vi "FPGA_HoppingScan_MultiRegion.vi"() -> ()   [LabVIEW 2024]
uses:
  <vilib>/Platform/TimedLoop/XDataNode/timing_clust.ctl
  <vilib>/Platform/TimedLoop/XDataNode/nitl_modes.ctl
  <vilib>/Platform/TimedLoop/XDataNode/wakeup.ctl
  <vilib>/rvi/FXPMathLib/FxpDiv/subVIs/nifxpmath_Div_SimConfig.ctl
  <vilib>/rvi/Emulation/niFpgaSctlEmulationGetInTimedLoop.vi
  <vilib>/rvi/Emulation/niFpgaProcessEmulError.vi
  <vilib>/rvi/eio/common/nirviEmuTemplateMethod_errors.vi
  <vilib>/rvi/Memory/Memory_Emulation/nirvimemoryFastEmulation.vi
  <vilib>/rvi/Memory/Memory_Emulation/nirvimemoryEmulation.vi
  <vilib>/rvi/Emulation/niFpgaEmulationIsFPGAContextNoSignature.vi
  <vilib>/rvi/DataTransferAndStorage/Container/Common/niFpgaContainerGetUniqueNameForEmu.vi
  <vilib>/rvi/errors/nirviReportUnexpectedCaseInternalError (U32).vi
  <vilib>/rvi/Emulation/niFpgaEmulationReportErrorSimple.vi
  <vilib>/rvi/Emulation/niFpgaGetClockAttributes.vi
  <vilib>/rvi/Emulation/niFpgaCriticalErrorInLSC.vi
  <vilib>/rvi/Memory/Memory_Emulation/niFpgaMemoryEmulationCacheClearOnFirstRun.vi
  <vilib>/rvi/Memory/Memory_Emulation/nirvimemoryEmulationManagerCache_MakeExclusive.vi
  <vilib>/rvi/Memory/Memory_Emulation/niFpgaMemoryEmulationValidateCache.vi
  <vilib>/rvi/Memory/Memory_Emulation/nirvimemoryEmulationManagerCache_InsertValue.vi
  <vilib>/Utility/error.llb/Clear Errors.vi
  <vilib>/rvi/Memory/Memory_Emulation/nirvimemoryEmulationManagerCache_ReleaseExclusive.vi
  <vilib>/rvi/Memory/Memory_Emulation/nirvimemoryEmulationManagerCache_GetValue.vi
  <vilib>/rvi/Memory/Memory_Emulation/nirvimemoryEmulationManagerCache_SetValue.vi
  <vilib>/rvi/FIFO/Fifo_Resource/nirvififoEmulationSetSize.vi
  <vilib>/rvi/FIFO/Fifo_Resource/nirviFifoEmulationQueueMgr.vi
  <instcachedir>/0/nirviFifoEmulationQueueMgr_E5CAEC123FF24DC58D834DCA3CDAA9B5.lvgen/nirviFifoEmulationQueueMgr_E5CAEC123FF24DC58D834DCA3CDAA9B5_001.vi
  <vilib>/rvi/errors/niFpgaSetErrorForExecOnDevCompSimple.vi
  <vilib>/rvi/eio/common/nirviEmuReportErrorAndStop.vi
  <vilib>/rvi/FIFO/Fifo_Resource/nirvififoEmulationCreateLock.vi
  <vilib>/rvi/FIFO/Fifo_Resource/nirvififoEmulationObtainLock.vi
  <vilib>/rvi/FIFO/Fifo_Resource/nirvififoEmulationReleaseLock.vi
  <vilib>/rvi/occurrence/nirviWaitOnOccurrenceBase.vi
  <vilib>/rvi/errors/nirviReportUnexpectedCaseInternalError.vi
  <vilib>/eio/utilities/niEioResolveVilibRelativePath.vi
  <vilib>/rvi/interface/RandomDataEmulation/niFpgaRandomDataHandleErrors.vi
  <vilib>/rvi/FXPMathLib/FxpDiv/simVIs/DllFxpDivTemp_sub.vi
  <vilib>/rvi/FIFO/Fifo_Resource/nirvififoEmulationDetermineInputValidOut.vi
  <vilib>/eio/EIONode/EIONode.xnode
  <vilib>/rvi/DataTransferAndStorage/Container/XNode/niFpgaContainer.xnode
  <vilib>/platform/TimedLoop/XDataNode/XDataNode.xnode
  <vilib>/rvi/DataTransferAndStorage/Register/Emulation/niFpgaRegisterEmulation.vi
  <vilib>/rvi/FIFO/Fifo_Resource/nirvififoEmulationGetNumberOfElementsToRead.vi
  <vilib>/rvi/FIFO/Fifo_Resource/nirvififoEmulationRead.vi
  <vilib>/rvi/interface/RandomDataEmulation/nirviRandomDataFpgaReadWriteTemplate.vi
  <vilib>/rvi/FXPMathLib/FxpSub/XNode/nifxpmath_Sub.xnode
  <vilib>/rvi/FXPMathLib/FxpAdd/XNode/nifxpmath_Add.xnode
  <vilib>/rvi/FXPMathLib/FxpMul/XNode/nifxpmath_Multiplier.xnode
  <vilib>/rvi/FXPMathLib/FxpDiv/XNode/nifxpmath_Div.xnode
  <vilib>/rvi/FIFO/Fifo_Resource/nirvififoEmulationWrite.vi
  <vilib>/rvi/FXPMathLib/sim/FxpSim.dll
  <vilib>/Platform/TimedLoop/XDataNode/XDNodeRunTimeDep.lvlib
panel:
  in  "LastScan":bool
  in  "InitScan":bool
  in  "DelayPoints":i32
  in  "Halting Threshold":fxp<+/-,48,16>
  out "point_scanned":u32
  in  "TotalPoints":u32
  in  "RetRate us":i32
  in  "AppRate_NF us":i32
  in  "AppRate_FF us":i32
  in  "Recording Threshold":fxp<+/-,48,16>
  in  "stop":bool
  out "TargetDone?":bool
  out "ScanFinished?":bool
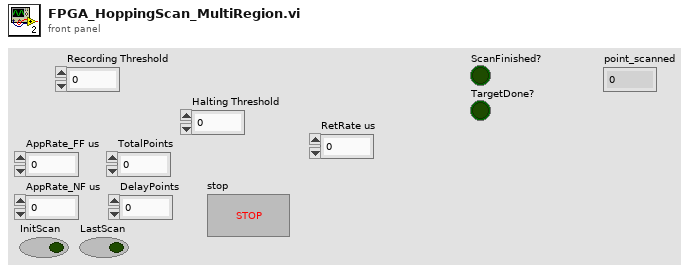
[diagram p1: front panel]
types:
  T1 = typedef "XDNodeRunTimeDep.lvlib/timing_clust.ctl" = cluster{"Expected End [f-1]":u64, "Actual End [f-1]":u64, "Finished Late? [f-1]":bool, "Expected End [i-1]":u64, "Actual End [i-1]":u64, "Finished Late? [i-1]":bool, "Expected Start [i]":u64, "Actual Start [i]":u64, "Expected Start [f]":u64, "Actual Start [f]":u64, "Source Name":string, "Structure Name":string, "Period":i64, "Deadline":i64, "Offset":i64, "Start":i64, "Priority":i32, "Timeout":i32, "Mode":T2, "Wakeup Reason":T3, "Error":errorcluster, "Source Type":string, "Secondary Source Type":string, "Global End Time":u64, "Global Start Time":u64, "Frame Duration":u64, "Iteration Duration":u64, "Assigned CPU":i32, "I/O Scan Engine Mode":u32}
  T2 = typedef "XDNodeRunTimeDep.lvlib/nitl_modes.ctl" = enum32{"No Change", "Process missed periods, maintain original phase", "Discard missed periods, maintain original phase", "Process missed periods, ignore original phase", "Discard missed periods, ignore original phase"}
  T3 = typedef "XDNodeRunTimeDep.lvlib/wakeup.ctl" = enum32{"Normal", "Aborted", "Asynchronous wakeup", "Timing source error", "Timed loop error", "Timeout"}
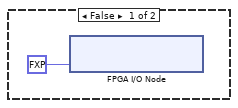
[diagram p2: hidden frame]
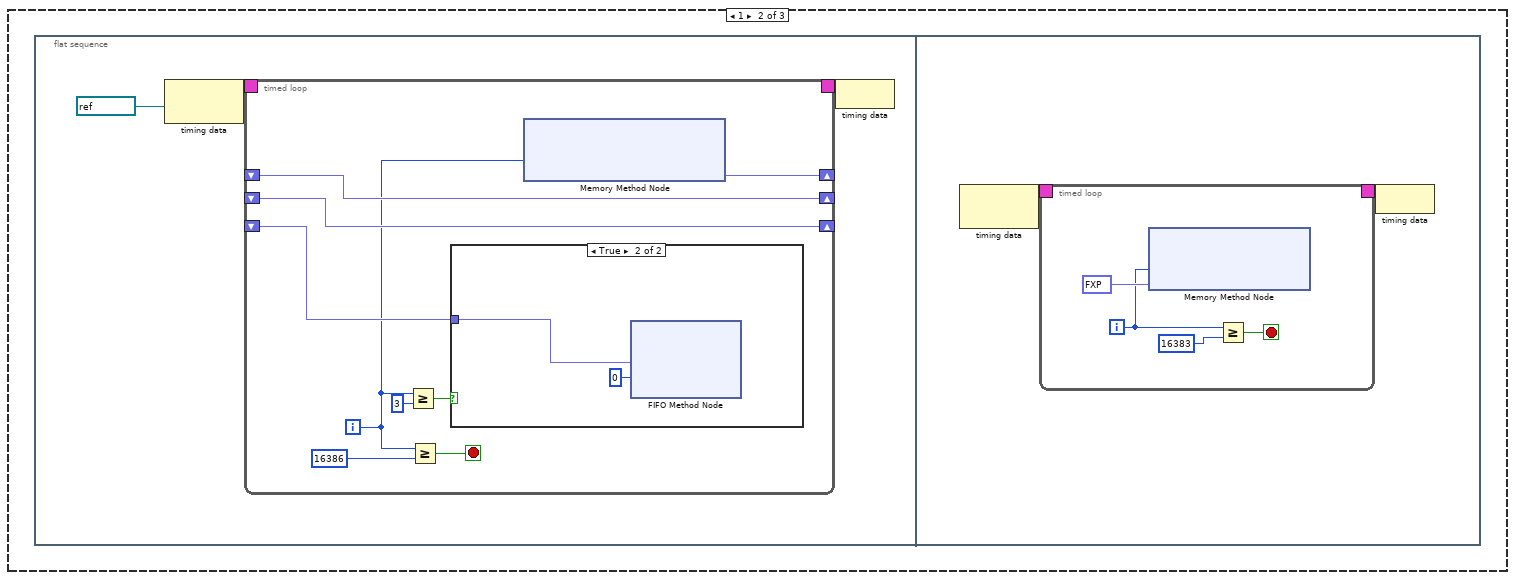
[diagram p5: hidden frame]
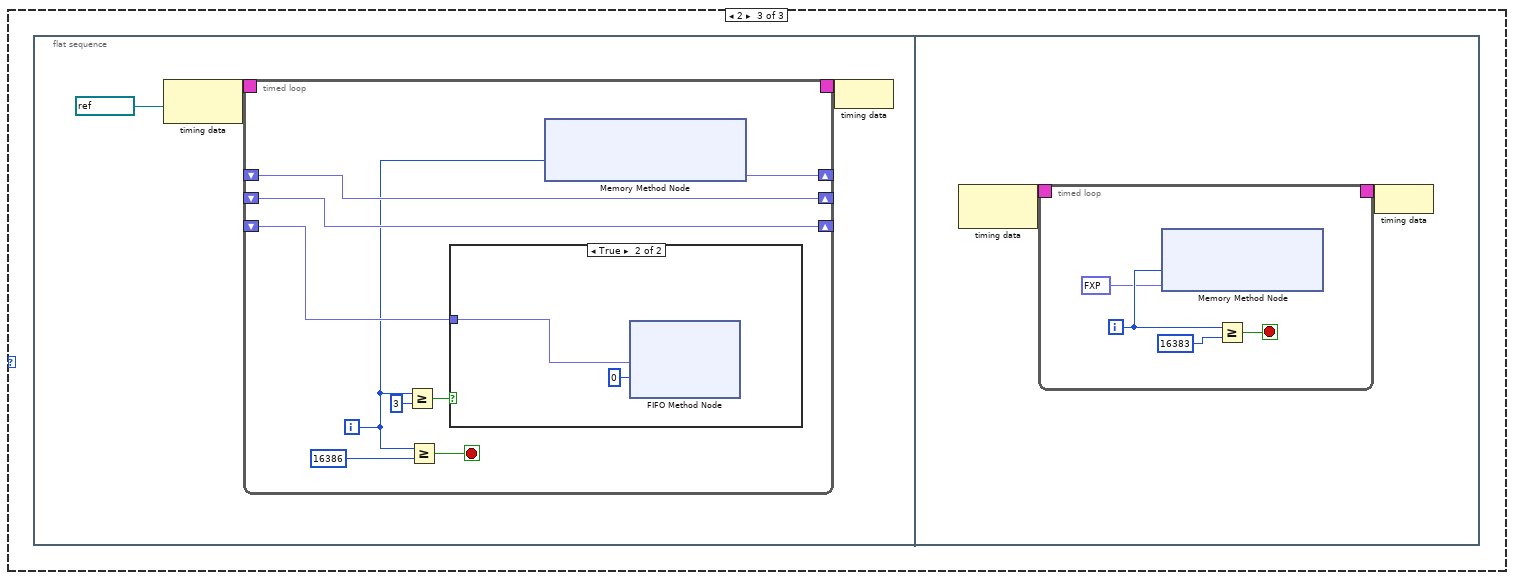
[diagram p7: hidden frame]
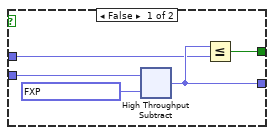
[diagram p14: hidden frame]
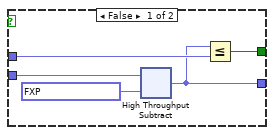
[diagram p15: hidden frame]
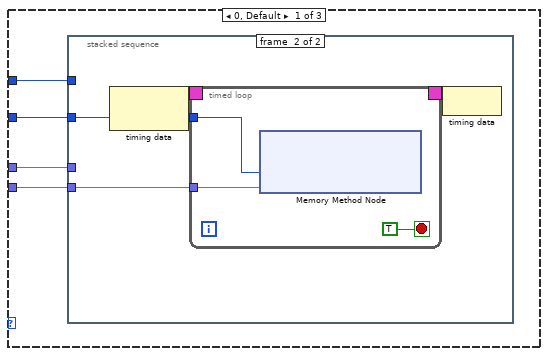
[diagram p17: hidden frame]
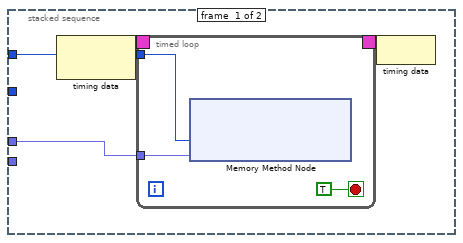
[diagram p18: hidden frame]
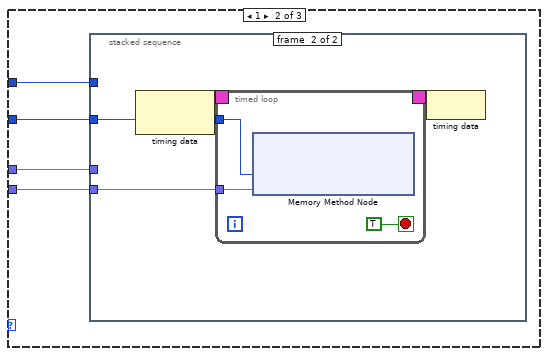
[diagram p19: hidden frame]
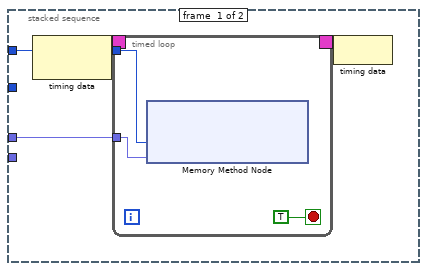
[diagram p20: hidden frame]
diagram:
  n1 = flat-sequence {
    tunnel: [w21] -> w1
    tunnel: w1 -> [w34]
    frame #0 {
      n2 = call "Wait18"("Count(mSec)"=u8 150) -> ()  [unwired: 1 out]
    }
    frame #1 {
      n3 = node-c288() -> (w5:T1)  [unwired: 1 in]
      n4 = timed-loop {
        timing: w5 -> [_]
        timing-out: [_] -> w4
        i -> [w14]
        stop <- w13 stop-if-true
        w16 = fxp<+/-,48,16> -100.0 ("Data")
        n5 = xnode ("Memory Method Node")("Address"=w14, "Data"=w16) -> ()  [unwired: 1 in, 1 out]
        n6 = xnode ("Memory Method Node")("Address"=w14, "Data"=w16) -> ()  [unwired: 1 in, 1 out]
        n7 = xnode ("Memory Method Node")("Address"=w14, "Data"=w16) -> ()  [unwired: 1 in, 1 out]
        n8 = Greater Or Equal?(x=w14, y=16383) -> (x >= y?=w13:bool)
      }
      n9 = case shown="True" "InitScan" {
        frame False {
          n10 = xnode "FPGA I/O Node"("Connector0/AO2"=fxp<+/-,20,5> 0.0 ("Connector0/AO0")) -> ()  [unwired: 1 in, 1 out]
        }
        frame True {
          w10 = fxp<+/-,20,5> 0.0 ("Connector0/AO0")
          n11 = for {
            N: 6 -> [_]
            i -> [w12]
            n12 = xnode ("Memory Method Node")("Address"=w12, "Data"=fxp<+/-,48,16> 0.0) -> ()  [unwired: 1 in, 1 out]
          }
          n13 = xnode "FPGA I/O Node"("Connector0/AO0"=w10, "Connector0/AO1"=w10, "Connector0/AO2"=w10) -> ()  [unwired: 3 in, 3 out]
        }
      }
      n14 = node-c288(w4) -> ()
      "ScanFinished?" <- FALSE
      "TargetDone?" <- FALSE
    }
    frame #2 {
      n15 = Generate Occurrence() -> (w21:refnum<k4>)
      n16 = call "Wait"("Count(mSec)"=u8 50) -> ()  [unwired: 1 out]
    }
    frame #3 {
      n17 = while {
        tunnel: w34 -> [w151]
        stop <- w153 stop-if-true
        n18 = xnode ("Register Read")() -> ("Data"=w154:bool)  [unwired: 1 in, 1 out]
        n19 = xnode ("FIFO Method Node")() -> ("Number of Elements to Read"=w157:u32)  [unwired: 1 in, 1 out]
        n20 = local read "ScanFinished?"() -> (w152:bool)
        n21 = Or(x=w154, y=w152) -> (x .or. y?=w153:bool)
        n22 = Greater Or Equal?(x=w157, y=u32 6) -> (x >= y?=w155:bool)
        n23 = case shown="True" w155 {
          tunnel: w151 -> [_ w158]
          frame False {
          }
          frame True {
            n24 = First Call?() -> (First Call?: T/F=w159:bool)
            n25 = case shown="True" w159 {
              tunnel: w158 -> [_ w160]
              frame False {
              }
              frame True {
                n26 = flat-sequence {
                  tunnel: [w163] -> w161
                  tunnel: w160 -> [w163]
                  tunnel: w161 -> [w164]
                  frame #0 {
                    n27 = call "Wait3"("Count(mSec)"=u8 4) -> ()  [unwired: 1 out]
                  }
                  frame #1 {
                    n28 = Set Occurrence(w164) -> ()
                  }
                }
              }
            }
          }
        }
      }
      n29 = while {
        tunnel: w34 -> [w136]
        stop <- w133 stop-if-true
        n30 = flat-sequence {
          tunnel: ["stop"] -> w138
          tunnel: w136 -> [w140]
          tunnel: [w140] -> w134
          tunnel: w138 -> [w143]
          tunnel: [w143] -> w137
          tunnel: [w142] -> w135
          tunnel: w134 -> [w142]
          tunnel: w137 -> [w147]
          tunnel: w135 -> [w146]
          tunnel: [w145] -> w133
          frame #0 {
            n31 = case shown="True" "stop" {
              tunnel: "stop" -> [_ w141]
              frame False {
              }
              frame True {
                n32 = xnode ("Register Write")("Data"=w141) -> ()  [unwired: 1 in, 1 out]
              }
            }
          }
          frame #1 {
            n33 = call "Wait2"("Count(uSec)"=u8 200) -> ()  [unwired: 1 out]
          }
          frame #2 {
            n34 = xnode ("Register Read")() -> ("Data"=w148:bool)  [unwired: 1 in, 1 out]
            n35 = local read "ScanFinished?"() -> (w149:bool)
            n36 = Compound Arithmetic op=OR(w149, w148, w147) -> (w145:bool)
            n37 = case shown="True" w145 {
              tunnel: w146 -> [_ w150]
              frame False {
              }
              frame True {
                n38 = Set Occurrence(w150) -> ()
              }
            }
          }
        }
      }
      n39 = flat-sequence {
        tunnel: w34 -> [w165]
        tunnel: [fxp<+/-,48,16> 0.0 ("Threshold")] -> w33
        tunnel: [w167] -> w31
        tunnel: [u8 0] -> w28
        tunnel: w33 -> [w170]
        tunnel: [w171] -> w32
        tunnel: w31 -> [w171]
        tunnel: [w170] -> w30
        tunnel: [w169] -> w29
        tunnel: w28 -> [w169]
        tunnel: w32 -> [w176]
        tunnel: w30 -> [w175]
        tunnel: w29 -> [w174]
        tunnel: [w173] -> w27
        tunnel: w27 -> [w1112]
        tunnel: [w1110] -> w26
        tunnel: [w1109] -> w24
        tunnel: w26 -> [w1124]
        tunnel: [w1124] -> w25
        tunnel: w24 -> [w1123]
        tunnel: [w1123] -> w23
        tunnel: w25 -> [w1129]
        tunnel: w23 -> [w1128]
        frame #0 {
          n40 = Wait on Occurrence(2:w165) -> ()  [unwired: 2 in, 1 out]
        }
        frame #1 {
          # "z piezo voltage"
          # "Swapchain indicator"
          n41 = xnode ("Register Read")() -> ("Data"=w167:bool)  [unwired: 1 in, 1 out]
        }
        frame #2 {
          n42 = call "Wait4"("Count(mSec)"=u8 4) -> ()  [unwired: 1 out]
        }
        frame #3 {
          n43 = case shown="False" w176 {
            tunnel: w175 -> [w179 w1108]
            tunnel: w174 -> [w178 _]
            tunnel: [w177 w1108] -> w173
            frame False {
              n44 = while {
                shift-right: [w186] -> w177
                shift-left: w179 -> [w213]
                shift-right: [w185] -> _
                shift-left: w178 -> [w196]
                stop <- w184 stop-if-true
                n45 = flat-sequence {
                  tunnel: w213 -> [w215]
                  tunnel: [w217] -> w212
                  tunnel: [w216] -> w208
                  tunnel: [w215] -> w200
                  tunnel: w196 -> [w214]
                  tunnel: [w214] -> w195
                  tunnel: w212 -> [w225]
                  tunnel: [w225] -> w211
                  tunnel: w208 -> [w224]
                  tunnel: [w224] -> w207
                  tunnel: w200 -> [w223]
                  tunnel: [w223] -> w199
                  tunnel: w195 -> [w222]
                  tunnel: [w222] -> w194
                  tunnel: w211 -> [w252]
                  tunnel: [w252] -> w210
                  tunnel: [w245] -> w209
                  tunnel: w207 -> [w251]
                  tunnel: [w251] -> w206
                  tunnel: [w246] -> w205
                  tunnel: [w249] -> w204
                  tunnel: [w248] -> w203
                  tunnel: [w247] -> w202
                  tunnel: w199 -> [w244]
                  tunnel: w194 -> [w250]
                  tunnel: [w250] -> w193
                  tunnel: [w241] -> w183
                  tunnel: [w243] -> w180
                  tunnel: [w289] -> w201
                  tunnel: [w288] -> w198
                  tunnel: [w287] -> w191
                  tunnel: [w286] -> w190
                  tunnel: [w285] -> w189
                  tunnel: [w284] -> w182
                  tunnel: w180 -> [w288]
                  tunnel: w183 -> [w284]
                  tunnel: w193 -> [w287]
                  tunnel: w202 -> [w285]
                  tunnel: w203 -> [w286]
                  tunnel: w204 -> [w289]
                  tunnel: w205 -> [w291]
                  tunnel: w206 -> [w290]
                  tunnel: w209 -> [w281]
                  tunnel: w210 -> [w280]
                  tunnel: w201 -> [w335]
                  tunnel: w198 -> [w334]
                  tunnel: [w334] -> w197
                  tunnel: [w333] -> w192
                  tunnel: w191 -> [w333]
                  tunnel: w190 -> [w332]
                  tunnel: w189 -> [w331]
                  tunnel: [w332] -> w188
                  tunnel: [w331] -> w187
                  tunnel: w182 -> [w330]
                  tunnel: [w330] -> w181
                  tunnel: w197 -> [w350]
                  tunnel: w192 -> [w349]
                  tunnel: w188 -> [w348]
                  tunnel: w187 -> [w347]
                  tunnel: [w346] -> w185
                  tunnel: [w345] -> w186
                  tunnel: [w344] -> w184
                  tunnel: w181 -> [w340]
                  frame #0 {
                    # "Data from target to host:\n0, 1: X, Y piezo voltage\n2, 3: X, Y piezo idx\n4: Z piezo voltage\n5: baseline current\n6: circular buffer pointer idx\n(7-8106): Z voltage\n(8107-16206): current"
                    # "Data from host to target:\n0, 1: X, Y piezo voltage\n2, 3: X, Y piezo idx\n4: distance (piezo voltage) to the last point\n5: retract height, \nall negative cases won't trigger approach of z piezo\nif -20, keep z and move xy\nif -30, full retract for z and move xy"
                    n46 = for {
                      N: 2 -> [_]
                      shift-right: [w221] -> w216
                      shift-left: _ -> [w219]
                      shift-right: [w219] -> w217
                      shift-left: _ -> [_]
                      i -> [w220]
                      n47 = xnode ("Memory Method Node")("Address"=w220) -> ("Data"=w221:fxp<+/-,48,16>)  [unwired: 1 in, 1 out]
                    }
                  }
                  frame #1 {
                    # "y"
                    # "x"
                    n48 = while {
                      shift-right: [w229] -> _
                      shift-left: i16 0 -> [w228]
                      stop <- w230 stop-if-true
                      n49 = xnode ("FIFO Method Node")("Timeout"=8192) -> ("Element"=w227:fxp<+/-,48,16>, "Timed Out?"=w234:bool)  [unwired: 1 in, 1 out]
                      n50 = Increment(x=w228) -> (x+1=w237:i16)
                      n51 = xnode ("Register Read")() -> ("Data"=w231:bool)  [unwired: 1 in, 1 out]
                      n52 = Select(t=w228, s=w234, f=w237) -> (s? t:f=w229:i16)
                      n53 = Not(x=w234) -> (.not. x?=w233:bool)
                      n54 = Equal?(x=w228, y=i16 5) -> (x = y?=w235:bool)
                      n55 = And(x=w235, y=w233) -> (x .and. y?=w232:bool)
                      n56 = xnode ("Memory Method Node")("Address"=w228, "Data"=w227) -> ()  [unwired: 1 in, 1 out]
                      n57 = Or(x=w232, y=w231) -> (x .or. y?=w230:bool)
                    }
                  }
                  frame #2 {
                    # "0"
                    # "5"
                    n58 = for {
                      N: 6 -> [_]
                      shift-right: [w278] -> w241
                      shift-left: _ -> [w277]
                      shift-right: [w277] -> w249
                      shift-left: _ -> [w276]
                      shift-right: [w276] -> w248
                      shift-left: _ -> [w275]
                      shift-right: [w275] -> w247
                      shift-left: _ -> [w274]
                      shift-right: [w274] -> w246
                      shift-left: _ -> [w273]
                      shift-right: [w273] -> w245
                      shift-left: _ -> [_]
                      i -> [w279]
                      n59 = xnode ("Memory Method Node")("Address"=w279) -> ("Data"=w278:fxp<+/-,48,16>)  [unwired: 1 in, 1 out]
                    }
                    n60 = Equal?(x=w241, y=fxp<+/-,48,16> -30.0) -> (x = y?=w240:bool)
                    n61 = case shown="True" w240 {
                      tunnel: w244 -> [w254 w258]
                      tunnel: [w254 w257] -> w243
                      tunnel: fxp<+/-,48,16> 0.0048828125 ("y") -> [_ w256]
                      frame False {
                      }
                      frame True {
                        n62 = flat-sequence {
                          tunnel: w258 -> [w261]
                          tunnel: w256 -> [w259]
                          tunnel: [w260] -> w255
                          tunnel: [w272] -> w257
                          tunnel: w255 -> [w272]
                          frame #0 {
                            n63 = while {
                              shift-right: [w265] -> w260
                              shift-left: w261 -> [w270]
                              tunnel: w259 -> [w264]
                              stop <- w266 stop-if-true
                              w267 = fxp<+/-,48,16> 0.0 ("y")
                              n64 = xnode "High Throughput Subtract"("x"=w270, "y"=w264) -> ("x-y"=w268:fxp<+/-,48,16>)
                              n65 = xnode ("Register Read")() -> ("Data"=w269:bool)  [unwired: 1 in, 1 out]
                              n66 = Less Or Equal?(x=w268, y=w267) -> (x <= y?=w262:bool)
                              n67 = Select(t=w267, s=w262, f=w268) -> (s? t:f=w265:fxp<+/-,48,16>)
                              n68 = local read "RetRate us"() -> (w263:i32)
                              n69 = xnode "FPGA I/O Node"("Connector0/AO2"=w265) -> ()  [unwired: 1 in, 1 out]
                              n70 = Compound Arithmetic op=OR(w262, w269) -> (w266:bool)
                              n71 = call "Wait10"("Count(uSec)"=w263) -> ()  [unwired: 1 out]
                            }
                          }
                          frame #1 {
                            n72 = call "Wait17"("Count(mSec)"=u16 2 ("Count(uSec)")) -> ()  [unwired: 1 out]
                          }
                        }
                      }
                    }
                  }
                  frame #3 {
                    n73 = xnode "High Throughput Subtract"("x"=w290, "y"=w291) -> ("x-y"=w293:fxp<+/-,48,16>)
                    n74 = xnode "High Throughput Subtract"("x"=w280, "y"=w281) -> ("x-y"=w283:fxp<+/-,48,16>)
                    n75 = Less Or Equal To 0?(x=w293) -> (x <= 0?=w292:bool)
                    n76 = Less Or Equal To 0?(x=w283) -> (x <= 0?=w282:bool)
                    n77 = while {
                      tunnel: w292 -> [w319]
                      tunnel: w291 -> [w318]
                      shift-right: [w312] -> _
                      shift-left: w290 -> [w314]
                      stop <- w315 stop-if-true
                      n78 = case shown="True" w319 {
                        tunnel: w318 -> [w321 w326]
                        tunnel: w314 -> [w323 w329]
                        tunnel: [w322 w327] -> w313
                        tunnel: [w320 w325] -> w312
                        frame False {
                          n79 = xnode "High Throughput Subtract"("x"=w323, "y"=fxp<+/-,48,16> 0.00030517578125) -> ("x-y"=w320:fxp<+/-,48,16>)
                          n80 = Less Or Equal?(x=w320, y=w321) -> (x <= y?=w322:bool)
                        }
                        frame True {
                          n81 = xnode ("High Throughput Add")("x"=w329, "y"=fxp<+/-,48,16> 0.00030517578125) -> ("x+y"=w325:fxp<+/-,48,16>)
                          n82 = Greater Or Equal?(x=w325, y=w326) -> (x >= y?=w327:bool)
                        }
                      }
                      n83 = call "Wait6"("Count(uSec)"=u32 70) -> ()  [unwired: 1 out]
                      n84 = xnode ("Register Read")() -> ("Data"=w316:bool)  [unwired: 1 in, 1 out]
                      n85 = xnode "FPGA I/O Node"("Connector0/AO1"=w312) -> ()  [unwired: 1 in, 1 out]
                      n86 = Or(x=w313, y=w316) -> (x .or. y?=w315:bool)
                    }
                    n87 = while {
                      tunnel: w282 -> [w301]
                      tunnel: w281 -> [w300]
                      shift-right: [w294] -> _
                      shift-left: w280 -> [w296]
                      stop <- w297 stop-if-true
                      n88 = case shown="True" w301 {
                        tunnel: w300 -> [w302 w307]
                        tunnel: w296 -> [w305 w311]
                        tunnel: [w304 w309] -> w295
                        tunnel: [w303 w308] -> w294
                        frame False {
                          n89 = xnode "High Throughput Subtract"("x"=w305, "y"=fxp<+/-,48,16> 0.00030517578125) -> ("x-y"=w303:fxp<+/-,48,16>)
                          n90 = Less Or Equal?(x=w303, y=w302) -> (x <= y?=w304:bool)
                        }
                        frame True {
                          n91 = xnode ("High Throughput Add")("x"=w311, "y"=fxp<+/-,48,16> 0.00030517578125) -> ("x+y"=w308:fxp<+/-,48,16>)
                          n92 = Greater Or Equal?(x=w308, y=w307) -> (x >= y?=w309:bool)
                        }
                      }
                      n93 = call "Wait5"("Count(uSec)"=u32 70) -> ()  [unwired: 1 out]
                      n94 = xnode ("Register Read")() -> ("Data"=w298:bool)  [unwired: 1 in, 1 out]
                      n95 = xnode "FPGA I/O Node"("Connector0/AO0"=w294) -> ()  [unwired: 1 in, 1 out]
                      n96 = Or(x=w295, y=w298) -> (x .or. y?=w297:bool)
                    }
                  }
                  frame #4 {
                    n97 = xnode ("High Throughput Multiply")("x"=w335, "y"=fxp<+/-,48,16> 1600.0) -> ("x*y"=w337:fxp<+/-,52,20>)
                    n98 = To Unsigned Long Integer(number=w337) -> (unsigned 32bit integer=w338:u32)
                    n99 = call "Wait7"("Count(uSec)"=w338) -> ()  [unwired: 1 out]
                  }
                  frame #5 {
                    # "Y, X idx"
                    n100 = xnode ("Register Read")() -> ("Data"=w343:bool)  [unwired: 1 in, 1 out]
                    n101 = Less Or Equal?(x=w340, y=fxp<+/-,48,16> -20.0) -> (x <= y?=w341:bool)
                    n102 = Or(x=w341, y=w343) -> (x .or. y?=w342:bool)
                    n103 = case shown="False" w342 {
                      tunnel: w350 -> [w370 w1107]
                      tunnel: w349 -> [w368 w1106]
                      tunnel: w348 -> [w362 _]
                      tunnel: w347 -> [w361 _]
                      tunnel: [w359 w1107] -> w345
                      tunnel: [w360 w1106] -> w346
                      tunnel: [w358 w1103] -> w344
                      tunnel: w341 -> [_ w1105]
                      tunnel: w340 -> [w354 _]
                      frame False {
                        n104 = flat-sequence {
                          tunnel: [w376] -> w373
                          tunnel: [w381] -> w372
                          tunnel: [w380] -> w371
                          tunnel: w370 -> [w379]
                          tunnel: [w379] -> w369
                          tunnel: w368 -> [w378]
                          tunnel: [w378] -> w367
                          tunnel: [0] -> w366
                          tunnel: [w376] -> w353
                          tunnel: [FALSE] -> w351
                          tunnel: w373 -> [w427]
                          tunnel: w372 -> [w426]
                          tunnel: w371 -> [w425]
                          tunnel: w369 -> [w424]
                          tunnel: w367 -> [w423]
                          tunnel: w366 -> [w418]
                          tunnel: [w422] -> w365
                          tunnel: [w421] -> w364
                          tunnel: [w420] -> w363
                          tunnel: w353 -> [w419]
                          tunnel: [w419] -> w352
                          tunnel: w351 -> [w417]
                          tunnel: w365 -> [w757]
                          tunnel: w364 -> [w759]
                          tunnel: w363 -> [w760]
                          tunnel: w362 -> [w762]
                          tunnel: w361 -> [w761]
                          tunnel: [w758] -> w357
                          tunnel: [w757] -> w356
                          tunnel: [w754] -> w355
                          tunnel: w352 -> [w753]
                          tunnel: [w1083] -> w358
                          tunnel: [w1082] -> w359
                          tunnel: [w1084] -> w360
                          tunnel: w357 -> [w1084]
                          tunnel: w356 -> [w1079]
                          tunnel: w355 -> [w1083]
                          tunnel: w354 -> [w1080]
                          frame #0 {
                            n105 = for {
                              N: 32 -> [_]
                              shift-right: [w414] -> w384
                              shift-left: fxp<+/-,48,16> 0.0 -> [w415]
                              n106 = xnode "FPGA I/O Node"() -> ("Connector0/AI3"=w416:fxp<+/-,27,5>)  [unwired: 1 in, 1 out]
                              n107 = xnode ("High Throughput Add")("x"=w416, "y"=w415) -> ("x+y"=w414:fxp<+/-,48,16>)
                            }
                            n108 = local read "Halting Threshold"() -> (w375:fxp<+/-,48,16>)
                            n109 = local read "Recording Threshold"() -> (w382:fxp<+/-,48,16>)
                            n110 = xnode "High Throughput Divide"("x"=w384, "y"=fxp<+/-,48,16> 32.0) -> ("x/y"=w376:fxp<+/-,48,16>)
                            n111 = xnode ("High Throughput Multiply")("x"=w376, "y"=w382) -> ("x*y"=w381:fxp<+/-,48,16>)
                            n112 = xnode ("High Throughput Multiply")("x"=w376, "y"=w375) -> ("x*y"=w380:fxp<+/-,48,16>)
                          }
                          frame #1 {
                            n113 = while {
                              tunnel: w427 -> [w490]
                              tunnel: w426 -> [w489]
                              tunnel: w425 -> [w488]
                              shift-right: [w467] -> w422
                              shift-left: w424 -> [w487]
                              shift-right: [w466] -> w421
                              shift-left: w423 -> [w486]
                              shift-right: [w449] -> _
                              shift-left: w418 -> [w485]
                              shift-right: [w450] -> _
                              shift-left: w418 -> [w474]
                              tunnel: [w460] -> w420
                              shift-right: [w434] -> _
                              shift-left: w418 -> [w438]
                              shift-right: [w428] -> _
                              shift-left: w417 -> [w432]
                              stop <- w463 stop-if-true
                              n114 = flat-sequence {
                                tunnel: w474 -> [w494]
                                tunnel: w485 -> [w495]
                                tunnel: w486 -> [w496]
                                tunnel: w487 -> [w497]
                                tunnel: w488 -> [w498]
                                tunnel: w489 -> [w499]
                                tunnel: w490 -> [w500]
                                tunnel: [w500] -> w459
                                tunnel: [w499] -> w458
                                tunnel: [w498] -> w457
                                tunnel: [w497] -> w456
                                tunnel: [w496] -> w455
                                tunnel: [w495] -> w454
                                tunnel: [w494] -> w453
                                tunnel: [w493] -> w452
                                tunnel: [w492] -> w439
                                tunnel: w438 -> [w492]
                                tunnel: [w491] -> w433
                                tunnel: w432 -> [w491]
                                tunnel: [w548] -> w484
                                tunnel: [w544] -> w483
                                tunnel: [w543] -> w482
                                tunnel: [w531] -> w478
                                tunnel: [w528] -> w477
                                tunnel: [w542] -> w473
                                tunnel: [w541] -> w471
                                tunnel: [w540] -> w468
                                tunnel: [w521] -> w465
                                tunnel: [w533] -> w461
                                tunnel: w459 -> [w555]
                                tunnel: w458 -> [w553]
                                tunnel: w457 -> [w523]
                                tunnel: w456 -> [w545]
                                tunnel: w455 -> [w541]
                                tunnel: w454 -> [w518]
                                tunnel: w453 -> [w542]
                                tunnel: w452 -> [w527]
                                tunnel: [w527] -> w451
                                tunnel: w439 -> [w507]
                                tunnel: [w508] -> w436
                                tunnel: w433 -> [w504]
                                tunnel: [w502] -> w431
                                tunnel: w484 -> [w627]
                                tunnel: w483 -> [w626]
                                tunnel: w482 -> [w628]
                                tunnel: [w628] -> w481
                                tunnel: [w627] -> w480
                                tunnel: [w626] -> w479
                                tunnel: w478 -> [w625]
                                tunnel: w477 -> [w624]
                                tunnel: [w625] -> w476
                                tunnel: [w624] -> w475
                                tunnel: w473 -> [w623]
                                tunnel: [w623] -> w472
                                tunnel: w471 -> [w622]
                                tunnel: [w622] -> w470
                                tunnel: [w621] -> w469
                                tunnel: w468 -> [w621]
                                tunnel: w465 -> [w620]
                                tunnel: [w620] -> w464
                                tunnel: [w619] -> w462
                                tunnel: w461 -> [w619]
                                tunnel: w451 -> [w618]
                                tunnel: [w618] -> w442
                                tunnel: [w617] -> w437
                                tunnel: w436 -> [w617]
                                tunnel: w431 -> [w616]
                                tunnel: [w616] -> w430
                                tunnel: w481 -> [w639]
                                tunnel: w480 -> [w650]
                                tunnel: w479 -> [w643]
                                tunnel: w476 -> [w645]
                                tunnel: w475 -> [w644]
                                tunnel: w472 -> [w631]
                                tunnel: w470 -> [w642]
                                tunnel: w469 -> [w633]
                                tunnel: w464 -> [w641]
                                tunnel: w462 -> [w640]
                                tunnel: [w650] -> w448
                                tunnel: [w646] -> w447
                                tunnel: [w643] -> w446
                                tunnel: [w642] -> w445
                                tunnel: [w641] -> w444
                                tunnel: [w640] -> w443
                                tunnel: w442 -> [w637]
                                tunnel: [w637] -> w441
                                tunnel: [w636] -> w440
                                tunnel: w437 -> [w635]
                                tunnel: [w635] -> w435
                                tunnel: w430 -> [w634]
                                tunnel: [w634] -> w429
                                tunnel: [w747] -> w460
                                tunnel: [w748] -> w463
                                tunnel: [w749] -> w466
                                tunnel: [w750] -> w467
                                tunnel: [w751] -> w450
                                tunnel: [w752] -> w449
                                tunnel: w448 -> [w752]
                                tunnel: w447 -> [w751]
                                tunnel: w446 -> [w750]
                                tunnel: w445 -> [w749]
                                tunnel: w444 -> [w748]
                                tunnel: w443 -> [w747]
                                tunnel: w441 -> [w745]
                                tunnel: w440 -> [w744]
                                tunnel: [w738] -> w434
                                tunnel: w435 -> [w738]
                                tunnel: w429 -> [w737]
                                tunnel: [w737] -> w428
                                frame #0 {
                                n115 = call "Tick Count"() -> ("Tick Count(uSec)"=w493:u32)
                                }
                                frame #1 {
                                w505 = 16
                                w520 = 1 ("y")
                                w546 = fxp<+/-,48,16> 0.0 ("y")
                                # "brake zone"
                                # "recording zone"
                                # "speed switch"
                                n116 = for {
                                N: w505 -> [_]
                                shift-right: [w613] -> w532
                                shift-left: w546 -> [w614]
                                shift-right: [w610] -> w530
                                shift-left: w546 -> [w612]
                                n117 = xnode "FPGA I/O Node"() -> ("Connector0/AI2"=w615:fxp<+/-,27,5>, "Connector0/AI3"=w611:fxp<+/-,27,5>)  [unwired: 2 in, 2 out]
                                n118 = xnode ("High Throughput Add")("x"=w612, "y"=w611) -> ("x+y"=w610:fxp<+/-,48,16>)
                                n119 = xnode ("High Throughput Add")("x"=w615, "y"=w614) -> ("x+y"=w613:fxp<+/-,48,16>)
                                }
                                n120 = To Fixed-Point(number=w505) -> (fixed-point=w529:fxp<+/-,48,16>)  [unwired: 1 in]
                                n121 = local read "DelayPoints"() -> (w501:i32)
                                n122 = Not Equal To 0?(x=w507) -> (x != 0?=w506:bool)
                                n123 = Greater Or Equal?(x=w507, y=w501) -> (x >= y?=w514:bool)
                                n124 = Select(t=fxp<+/-,48,16> 0.0 ("y"), s=w506, f=fxp<+/-,48,16> 0.00030517578125 ("y")) -> (s? t:f=w515:fxp<+/-,48,16>)
                                n125 = xnode "High Throughput Divide"("x"=w532, "y"=w529) -> ("x/y"=w531:fxp<+/-,48,16>)
                                n126 = xnode "High Throughput Divide"("x"=w530, "y"=w529) -> ("x/y"=w528:fxp<+/-,48,16>)
                                n127 = xnode ("High Throughput Add")("x"=w515, "y"=w545) -> ("x+y"=w534:fxp<+/-,48,16>)
                                n128 = xnode "High Throughput Subtract"("x"=w555, "y"=w528) -> ("x-y"=w554:fxp<+/-,48,16>)
                                n129 = Absolute Value(x=w554) -> (abs(x)=w524:fxp<+,48,16>)
                                n130 = Less Or Equal?(x=w534, y=fxp<+/-,48,16> 9.75) -> (x <= y?=w536:bool)
                                n131 = Greater Or Equal?(x=w534, y=fxp<+/-,48,16> -0.125) -> (x >= y?=w537:bool)
                                n132 = And(x=w537, y=w536) -> (x .and. y?=w535:bool)
                                n133 = Greater Or Equal?(x=w524, y=w553) -> (x >= y?=w552:bool)
                                n134 = Less Or Equal?(x=w524, y=w523) -> (x <= y?=w526:bool)
                                n135 = Increment(x=w518) -> (x+1=w551:i32)
                                n136 = Select(t=w551, s=w552, f=0) -> (s? t:f=w548:i32)
                                n137 = xnode ("Register Read")() -> ("Data"=w540:bool)  [unwired: 1 in, 1 out]
                                n138 = Greater Or Equal?(x=w548, y=w520) -> (x >= y?=w503:bool)
                                n139 = Equal?(x=w548, y=0 ("f")) -> (x = y?=w547:bool)
                                n140 = Not(x=w526) -> (.not. x?=w533:bool)
                                n141 = Or(x=w504, y=w503) -> (x .or. y?=w502:bool)
                                n142 = Select(t=1 ("y"), s=w502, f=0) -> (s? t:f=w510:i32)
                                n143 = Add(x=w507, y=w510) -> (x+y=w509:i32)
                                n144 = Select(t=0, s=w514, f=w509) -> (s? t:f=w508:i32)
                                n145 = Greater Or Equal?(x=w548, y=w520) -> (x >= y?=w543:bool)
                                n146 = Compound Arithmetic op=AND(w526, invert w540, w535) -> (w522:bool)
                                n147 = Or(x=w547, y=w502) -> (x .or. y?=w519:bool)
                                n148 = And(x=w519, y=w522) -> (x .and. y?=w525:bool)
                                n149 = Not(x=w522) -> (.not. x?=w521:bool)
                                n150 = Select(t=w534, s=w525, f=w545) -> (s? t:f=w544:fxp<+/-,48,16>)
                                }
                                frame #2 {
                                n151 = xnode "FPGA I/O Node"("Connector0/AO2"=w626) -> ()  [unwired: 1 in, 1 out]
                                }
                                frame #3 {
                                n152 = Not(x=w633) -> (.not. x?=w632:bool)
                                n153 = Less?(x=w631, y=8099 ("f")) -> (x < y?=w629:bool)
                                n154 = case shown="True" w632 {
                                tunnel: w642 -> [_ w658]
                                tunnel: w631 -> [_ w654]
                                tunnel: w645 -> [_ w652]
                                tunnel: w644 -> [_ w651]
                                frame False {
                                }
                                frame True {
                                n155 = Add(x=w654, y=7) -> (x+y=w656:i32)
                                n156 = Add(x=w654, y=8107) -> (x+y=w653:i32)
                                n157 = case shown="2" w658 {
                                tunnel: w656 -> [w662 w686 w714]
                                tunnel: w653 -> [w661 w685 w713]
                                tunnel: w652 -> [w660 w687 w712]
                                tunnel: w651 -> [w659 w688 w711]
                                frame 0, Default {
                                n158 = stacked-sequence {
                                tunnel: w662 -> [w666 _]
                                tunnel: w661 -> [_ w677]
                                tunnel: w660 -> [w665 _]
                                tunnel: w659 -> [_ w676]
                                frame #0 {
                                n159 = node-c288() -> (w664:T1)  [unwired: 1 in]
                                n160 = timed-loop {
                                timing: w664 -> [_]
                                timing-out: [_] -> w663
                                tunnel: w666 -> [w669]
                                tunnel: w665 -> [w668]
                                stop <- TRUE stop-if-true
                                n161 = xnode ("Memory Method Node")("Address"=w669, "Data"=w668) -> ()  [unwired: 1 in, 1 out]
                                }
                                n162 = node-c288(w663) -> ()
                                }
                                frame #1 {
                                n163 = node-c288() -> (w675:T1)  [unwired: 1 in]
                                n164 = timed-loop {
                                timing: w675 -> [_]
                                timing-out: [_] -> w674
                                tunnel: w677 -> [w680]
                                tunnel: w676 -> [w679]
                                stop <- TRUE stop-if-true
                                n165 = xnode ("Memory Method Node")("Address"=w680, "Data"=w679) -> ()  [unwired: 1 in, 1 out]
                                }
                                n166 = node-c288(w674) -> ()
                                }
                                }
                                }
                                frame 1 {
                                n167 = stacked-sequence {
                                tunnel: w688 -> [_ w703]
                                tunnel: w687 -> [w692 _]
                                tunnel: w686 -> [w691 _]
                                tunnel: w685 -> [_ w702]
                                frame #0 {
                                n168 = node-c288() -> (w690:T1)  [unwired: 1 in]
                                n169 = timed-loop {
                                timing: w690 -> [_]
                                timing-out: [_] -> w689
                                tunnel: w692 -> [w695]
                                tunnel: w691 -> [w694]
                                stop <- TRUE stop-if-true
                                n170 = xnode ("Memory Method Node")("Address"=w694, "Data"=w695) -> ()  [unwired: 1 in, 1 out]
                                }
                                n171 = node-c288(w689) -> ()
                                }
                                frame #1 {
                                n172 = node-c288() -> (w701:T1)  [unwired: 1 in]
                                n173 = timed-loop {
                                timing: w701 -> [_]
                                timing-out: [_] -> w700
                                tunnel: w703 -> [w706]
                                tunnel: w702 -> [w705]
                                stop <- TRUE stop-if-true
                                n174 = xnode ("Memory Method Node")("Address"=w705, "Data"=w706) -> ()  [unwired: 1 in, 1 out]
                                }
                                n175 = node-c288(w700) -> ()
                                }
                                }
                                }
                                frame 2 {
                                n176 = stacked-sequence {
                                tunnel: w711 -> [_ w729]
                                tunnel: w712 -> [w718 _]
                                tunnel: w714 -> [w717 _]
                                tunnel: w713 -> [_ w728]
                                frame #0 {
                                n177 = node-c288() -> (w716:T1)  [unwired: 1 in]
                                n178 = timed-loop {
                                timing: w716 -> [_]
                                timing-out: [_] -> w715
                                tunnel: w718 -> [w719]
                                tunnel: w717 -> [w720]
                                stop <- TRUE stop-if-true
                                n179 = xnode ("Memory Method Node")("Address"=w720, "Data"=w719) -> ()  [unwired: 1 in, 1 out]
                                }
                                n180 = node-c288(w715) -> ()
                                }
                                frame #1 {
                                n181 = node-c288() -> (w727:T1)  [unwired: 1 in]
                                n182 = timed-loop {
                                timing: w727 -> [_]
                                timing-out: [_] -> w726
                                tunnel: w729 -> [w730]
                                tunnel: w728 -> [w731]
                                stop <- TRUE stop-if-true
                                n183 = xnode ("Memory Method Node")("Address"=w731, "Data"=w730) -> ()  [unwired: 1 in, 1 out]
                                }
                                n184 = node-c288(w726) -> ()
                                }
                                }
                                }
                                }
                                }
                                }
                                n185 = local read "AppRate_NF us"() -> (w649:i32)
                                n186 = local read "AppRate_FF us"() -> (w648:i32)
                                n187 = Increment(x=w631) -> (x+1=w647:i32)
                                n188 = Select(t=w649, s=w639, f=w648) -> (s? t:f=w636:i32)
                                n189 = Select(t=w647, s=w629, f=0) -> (s? t:f=w646:i32)
                                }
                                frame #4 {
                                n190 = call "Tick Count2"() -> ("Tick Count(uSec)"=w746:u32)
                                n191 = Subtract(x=w746, y=w745) -> (x-y=w743:i32)
                                n192 = Subtract(x=w744, y=w743) -> (x-y=w742:i32)
                                n193 = In Range and Coerce(upper limit=80000, x=w742, lower limit=1) -> (coerced(x)=w739:i32)  [unwired: 1 out]
                                n194 = call "Wait9"("Count(uSec)"=w739) -> ()  [unwired: 1 out]
                                }
                              }
                            }
                          }
                          frame #2 {
                            n195 = xnode ("Register Read")() -> ("Data"=w756:bool)  [unwired: 1 in, 1 out]
                            n196 = Compound Arithmetic op=AND(w760, invert w756) -> (w763:bool)
                            n197 = case shown="True" w763 {
                              tunnel: w762 -> [_ w783]
                              tunnel: w761 -> [_ w784]
                              tunnel: w759 -> [w765 w782]
                              tunnel: [w765 w781] -> w758
                              tunnel: [FALSE w777] -> w755
                              tunnel: w753 -> [_ w776]
                              frame False {
                              }
                              frame True {
                                w785 = fxp<+/-,48,16> 0.0 ("ZPeizoOffset")
                                n198 = for {
                                N: 16 -> [_]
                                shift-right: [w1071] -> w774
                                shift-left: w785 -> [w1075]
                                shift-right: [w1070] -> w771
                                shift-left: w785 -> [w1073]
                                shift-right: [w1067] -> w768
                                shift-left: w785 -> [w1069]
                                n199 = xnode "FPGA I/O Node"() -> ("Connector0/AI0"=w1074:fxp<+/-,27,5>, "Connector0/AI1"=w1072:fxp<+/-,27,5>, "Connector0/AI2"=w1068:fxp<+/-,27,5>)  [unwired: 3 in, 3 out]
                                n200 = xnode ("High Throughput Add")("x"=w1074, "y"=w1075) -> ("x+y"=w1071:fxp<+/-,48,16>)
                                n201 = xnode ("High Throughput Add")("x"=w1069, "y"=w1068) -> ("x+y"=w1067:fxp<+/-,48,16>)
                                n202 = xnode ("High Throughput Add")("x"=w1072, "y"=w1073) -> ("x+y"=w1070:fxp<+/-,48,16>)
                                }
                                n203 = feedback #1(u32 0 ("Timeout")) -> (w779:u32)
                                n204 = Increment(x=w779) -> (x+1=w766:u32)
                                "point_scanned" <- w766
                                n205 = feedback-in #1(w766) -> ()
                                n206 = local read "TotalPoints"() -> (w778:u32)
                                n207 = Greater Or Equal?(x=w766, y=w778) -> (x >= y?=w777:bool)
                                n208 = xnode "High Throughput Divide"("x"=w771, "y"=fxp<+/-,48,16> 16.0 ("ZPeizoOffset")) -> ("x/y"=w770:fxp<+/-,48,16>)
                                n209 = xnode "High Throughput Divide"("x"=w774, "y"=fxp<+/-,48,16> 16.0 ("ZPeizoOffset")) -> ("x/y"=w773:fxp<+/-,48,16>)
                                n210 = xnode "High Throughput Divide"("x"=w768, "y"=fxp<+/-,48,16> 16.0 ("ZPeizoOffset")) -> ("x/y"=w767:fxp<+/-,48,16>)
                                n211 = stacked-sequence {
                                tunnel: w773 -> [w868 _ _ _ _ _ _]
                                tunnel: w770 -> [_ w900 _ _ _ _ _]
                                tunnel: w767 -> [_ _ _ _ w996 _ _]
                                tunnel: w784 -> [_ _ w933 _ _ _ _]
                                tunnel: w783 -> [_ _ _ w965 _ _ _]
                                tunnel: w782 -> [w869 w901 w932 w964 w997 w1029 w1064]
                                tunnel: [_ _ _ _ _ _ w1062] -> w781
                                tunnel: w776 -> [_ _ _ _ _ w1028 _]
                                frame #0 {
                                n212 = case shown="2" w869 {
                                tunnel: w868 -> [w872 w882 w890]
                                frame 0, Default {
                                n213 = node-c288() -> (w871:T1)  [unwired: 1 in]
                                n214 = timed-loop {
                                timing: w871 -> [_]
                                timing-out: [_] -> w870
                                tunnel: w872 -> [w874]
                                stop <- TRUE stop-if-true
                                n215 = xnode ("Memory Method Node")("Address"=u32 0, "Data"=w874) -> ()  [unwired: 1 in, 1 out]
                                }
                                n216 = node-c288(w870) -> ()
                                }
                                frame 1 {
                                n217 = node-c288() -> (w881:T1)  [unwired: 1 in]
                                n218 = timed-loop {
                                timing: w881 -> [_]
                                timing-out: [_] -> w880
                                tunnel: w882 -> [w884]
                                stop <- TRUE stop-if-true
                                n219 = xnode ("Memory Method Node")("Address"=u32 0, "Data"=w884) -> ()  [unwired: 1 in, 1 out]
                                }
                                n220 = node-c288(w880) -> ()
                                }
                                frame 2 {
                                n221 = node-c288() -> (w892:T1)  [unwired: 1 in]
                                n222 = timed-loop {
                                timing: w892 -> [_]
                                timing-out: [_] -> w891
                                tunnel: w890 -> [w893]
                                stop <- TRUE stop-if-true
                                n223 = xnode ("Memory Method Node")("Address"=u32 0, "Data"=w893) -> ()  [unwired: 1 in, 1 out]
                                }
                                n224 = node-c288(w891) -> ()
                                }
                                }
                                }
                                frame #1 {
                                n225 = case shown="2" w901 {
                                tunnel: w900 -> [w904 w914 w922]
                                frame 0, Default {
                                n226 = node-c288() -> (w903:T1)  [unwired: 1 in]
                                n227 = timed-loop {
                                timing: w903 -> [_]
                                timing-out: [_] -> w902
                                tunnel: w904 -> [w906]
                                stop <- TRUE stop-if-true
                                n228 = xnode ("Memory Method Node")("Address"=u32 1, "Data"=w906) -> ()  [unwired: 1 in, 1 out]
                                }
                                n229 = node-c288(w902) -> ()
                                }
                                frame 1 {
                                n230 = node-c288() -> (w913:T1)  [unwired: 1 in]
                                n231 = timed-loop {
                                timing: w913 -> [_]
                                timing-out: [_] -> w912
                                tunnel: w914 -> [w916]
                                stop <- TRUE stop-if-true
                                n232 = xnode ("Memory Method Node")("Address"=u32 1, "Data"=w916) -> ()  [unwired: 1 in, 1 out]
                                }
                                n233 = node-c288(w912) -> ()
                                }
                                frame 2 {
                                n234 = node-c288() -> (w924:T1)  [unwired: 1 in]
                                n235 = timed-loop {
                                timing: w924 -> [_]
                                timing-out: [_] -> w923
                                tunnel: w922 -> [w925]
                                stop <- TRUE stop-if-true
                                n236 = xnode ("Memory Method Node")("Address"=u32 0, "Data"=w925) -> ()  [unwired: 1 in, 1 out]
                                }
                                n237 = node-c288(w923) -> ()
                                }
                                }
                                }
                                frame #2 {
                                n238 = case shown="2" w932 {
                                tunnel: w933 -> [w936 w946 w954]
                                frame 0, Default {
                                n239 = node-c288() -> (w935:T1)  [unwired: 1 in]
                                n240 = timed-loop {
                                timing: w935 -> [_]
                                timing-out: [_] -> w934
                                tunnel: w936 -> [w938]
                                stop <- TRUE stop-if-true
                                n241 = xnode ("Memory Method Node")("Address"=u32 2, "Data"=w938) -> ()  [unwired: 1 in, 1 out]
                                }
                                n242 = node-c288(w934) -> ()
                                }
                                frame 1 {
                                n243 = node-c288() -> (w945:T1)  [unwired: 1 in]
                                n244 = timed-loop {
                                timing: w945 -> [_]
                                timing-out: [_] -> w944
                                tunnel: w946 -> [w948]
                                stop <- TRUE stop-if-true
                                n245 = xnode ("Memory Method Node")("Address"=u32 2, "Data"=w948) -> ()  [unwired: 1 in, 1 out]
                                }
                                n246 = node-c288(w944) -> ()
                                }
                                frame 2 {
                                n247 = node-c288() -> (w956:T1)  [unwired: 1 in]
                                n248 = timed-loop {
                                timing: w956 -> [_]
                                timing-out: [_] -> w955
                                tunnel: w954 -> [w957]
                                stop <- TRUE stop-if-true
                                n249 = xnode ("Memory Method Node")("Address"=u32 0, "Data"=w957) -> ()  [unwired: 1 in, 1 out]
                                }
                                n250 = node-c288(w955) -> ()
                                }
                                }
                                }
                                frame #3 {
                                n251 = case shown="2" w964 {
                                tunnel: w965 -> [w968 w978 w986]
                                frame 0, Default {
                                n252 = node-c288() -> (w967:T1)  [unwired: 1 in]
                                n253 = timed-loop {
                                timing: w967 -> [_]
                                timing-out: [_] -> w966
                                tunnel: w968 -> [w970]
                                stop <- TRUE stop-if-true
                                n254 = xnode ("Memory Method Node")("Address"=u32 3, "Data"=w970) -> ()  [unwired: 1 in, 1 out]
                                }
                                n255 = node-c288(w966) -> ()
                                }
                                frame 1 {
                                n256 = node-c288() -> (w977:T1)  [unwired: 1 in]
                                n257 = timed-loop {
                                timing: w977 -> [_]
                                timing-out: [_] -> w976
                                tunnel: w978 -> [w980]
                                stop <- TRUE stop-if-true
                                n258 = xnode ("Memory Method Node")("Address"=u32 3, "Data"=w980) -> ()  [unwired: 1 in, 1 out]
                                }
                                n259 = node-c288(w976) -> ()
                                }
                                frame 2 {
                                n260 = node-c288() -> (w988:T1)  [unwired: 1 in]
                                n261 = timed-loop {
                                timing: w988 -> [_]
                                timing-out: [_] -> w987
                                tunnel: w986 -> [w989]
                                stop <- TRUE stop-if-true
                                n262 = xnode ("Memory Method Node")("Address"=u32 0, "Data"=w989) -> ()  [unwired: 1 in, 1 out]
                                }
                                n263 = node-c288(w987) -> ()
                                }
                                }
                                }
                                frame #4 {
                                n264 = case shown="2" w997 {
                                tunnel: w996 -> [w1000 w1010 w1018]
                                frame 0, Default {
                                n265 = node-c288() -> (w999:T1)  [unwired: 1 in]
                                n266 = timed-loop {
                                timing: w999 -> [_]
                                timing-out: [_] -> w998
                                tunnel: w1000 -> [w1002]
                                stop <- TRUE stop-if-true
                                n267 = xnode ("Memory Method Node")("Address"=u32 4, "Data"=w1002) -> ()  [unwired: 1 in, 1 out]
                                }
                                n268 = node-c288(w998) -> ()
                                }
                                frame 1 {
                                n269 = node-c288() -> (w1009:T1)  [unwired: 1 in]
                                n270 = timed-loop {
                                timing: w1009 -> [_]
                                timing-out: [_] -> w1008
                                tunnel: w1010 -> [w1012]
                                stop <- TRUE stop-if-true
                                n271 = xnode ("Memory Method Node")("Address"=u32 4, "Data"=w1012) -> ()  [unwired: 1 in, 1 out]
                                }
                                n272 = node-c288(w1008) -> ()
                                }
                                frame 2 {
                                n273 = node-c288() -> (w1020:T1)  [unwired: 1 in]
                                n274 = timed-loop {
                                timing: w1020 -> [_]
                                timing-out: [_] -> w1019
                                tunnel: w1018 -> [w1021]
                                stop <- TRUE stop-if-true
                                n275 = xnode ("Memory Method Node")("Address"=u32 0, "Data"=w1021) -> ()  [unwired: 1 in, 1 out]
                                }
                                n276 = node-c288(w1019) -> ()
                                }
                                }
                                }
                                frame #5 {
                                n277 = case shown="2" w1029 {
                                tunnel: w1028 -> [w1032 w1042 w1050]
                                frame 0, Default {
                                n278 = node-c288() -> (w1031:T1)  [unwired: 1 in]
                                n279 = timed-loop {
                                timing: w1031 -> [_]
                                timing-out: [_] -> w1030
                                tunnel: w1032 -> [w1034]
                                stop <- TRUE stop-if-true
                                n280 = xnode ("Memory Method Node")("Address"=u32 5, "Data"=w1034) -> ()  [unwired: 1 in, 1 out]
                                }
                                n281 = node-c288(w1030) -> ()
                                }
                                frame 1 {
                                n282 = node-c288() -> (w1041:T1)  [unwired: 1 in]
                                n283 = timed-loop {
                                timing: w1041 -> [_]
                                timing-out: [_] -> w1040
                                tunnel: w1042 -> [w1044]
                                stop <- TRUE stop-if-true
                                n284 = xnode ("Memory Method Node")("Address"=u32 5, "Data"=w1044) -> ()  [unwired: 1 in, 1 out]
                                }
                                n285 = node-c288(w1040) -> ()
                                }
                                frame 2 {
                                n286 = node-c288() -> (w1052:T1)  [unwired: 1 in]
                                n287 = timed-loop {
                                timing: w1052 -> [_]
                                timing-out: [_] -> w1051
                                tunnel: w1050 -> [w1053]
                                stop <- TRUE stop-if-true
                                n288 = xnode ("Memory Method Node")("Address"=u32 0, "Data"=w1053) -> ()  [unwired: 1 in, 1 out]
                                }
                                n289 = node-c288(w1051) -> ()
                                }
                                }
                                }
                                frame #6 {
                                n290 = xnode ("FIFO Method Node")("Element"=w1064, "Timeout"=0) -> ()  [unwired: 1 in, 2 out]
                                n291 = Increment(x=w1064) -> (x+1=w1063:u8)
                                n292 = Greater Or Equal?(x=w1063, y=u8 3) -> (x >= y?=w1065:bool)
                                n293 = Select(t=w1064, s=w1065, f=u8 0) -> (s? t:f=w1062:u8)
                                }
                                }
                              }
                            }
                            n294 = Or(x=w756, y=w755) -> (x .or. y?=w754:bool)
                          }
                          frame #3 {
                            n295 = xnode ("Register Read")() -> ("Data"=w1078:bool)  [unwired: 1 in, 1 out]
                            n296 = Less Or Equal To 0?(x=w1079) -> (x <= 0?=w1077:bool)
                            n297 = Or(x=w1078, y=w1077) -> (x .or. y?=w1076:bool)
                            n298 = case shown="False" w1076 {
                              tunnel: w1079 -> [w1087 w1101]
                              tunnel: [w1089 w1101] -> w1082
                              tunnel: fxp<+/-,48,16> 0.0048828125 ("y") -> [w1088 _]
                              tunnel: w1080 -> [w1085 _]
                              frame False {
                                n299 = xnode "High Throughput Subtract"("x"=w1087, "y"=w1085) -> ("x-y"=w1086:fxp<+/-,48,16>)
                                n300 = while {
                                shift-right: [w1094] -> w1089
                                shift-left: w1087 -> [w1100]
                                tunnel: w1088 -> [w1093]
                                tunnel: w1086 -> [w1092]
                                stop <- w1095 stop-if-true
                                n301 = xnode "High Throughput Subtract"("x"=w1100, "y"=w1093) -> ("x-y"=w1096:fxp<+/-,48,16>)
                                n302 = xnode ("Register Read")() -> ("Data"=w1099:bool)  [unwired: 1 in, 1 out]
                                n303 = Less Or Equal To 0?(x=w1096) -> (x <= 0?=w1097:bool)
                                n304 = Less Or Equal?(x=w1096, y=w1092) -> (x <= y?=w1098:bool)
                                n305 = Select(t=fxp<+/-,48,16> 0.0, s=w1097, f=w1096) -> (s? t:f=w1094:fxp<+/-,48,16>)
                                n306 = local read "RetRate us"() -> (w1090:i32)
                                n307 = xnode "FPGA I/O Node"("Connector0/AO2"=w1094) -> ()  [unwired: 1 in, 1 out]
                                n308 = Compound Arithmetic op=OR(w1097, w1098, w1099) -> (w1095:bool)
                                n309 = call "Wait11"("Count(uSec)"=w1090) -> ()  [unwired: 1 out]
                                }
                              }
                              frame True {
                              }
                            }
                          }
                        }
                      }
                      frame True {
                        n310 = xnode ("Register Read")() -> ("Data"=w1102:bool)  [unwired: 1 in, 1 out]
                        n311 = Not(x=w1105) -> (.not. x?=w1104:bool)
                        n312 = Or(x=w1104, y=w1102) -> (x .or. y?=w1103:bool)
                      }
                    }
                  }
                }
              }
            }
            frame True {
            }
          }
        }
        frame #4 {
          n313 = while {
            shift-right: [w1116] -> _
            shift-left: w1112 -> [w1121]
            tunnel: fxp<+/-,48,16> 0.0048828125 ("y") -> [w1115]
            stop <- w1117 stop-if-true
            w1113 = fxp<+/-,48,16> 0.0 ("t")
            n314 = xnode "High Throughput Subtract"("x"=w1121, "y"=w1115) -> ("x-y"=w1118:fxp<+/-,48,16>)
            n315 = Less Or Equal To 0?(x=w1118) -> (x <= 0?=w1119:bool)
            n316 = Less Or Equal?(x=w1118, y=w1113) -> (x <= y?=w1120:bool)
            n317 = Select(t=w1113, s=w1119, f=w1118) -> (s? t:f=w1116:fxp<+/-,48,16>)
            n318 = local read "RetRate us"() -> (w1114:i32)
            n319 = xnode "FPGA I/O Node"("Connector0/AO2"=w1116) -> ()  [unwired: 1 in, 1 out]
            n320 = Compound Arithmetic op=OR(w1119, w1120) -> (w1117:bool)
            n321 = call "Wait12"("Count(uSec)"=w1114) -> ()  [unwired: 1 out]
          }
          n322 = xnode "FPGA I/O Node"() -> ("Connector0/AI0"=w1110:fxp<+/-,27,5>, "Connector0/AI1"=w1109:fxp<+/-,27,5>)  [unwired: 2 in, 2 out]
        }
        frame #5 {
          n323 = call "Wait15"("Count(uSec)"=u8 100) -> ()  [unwired: 1 out]
        }
        frame #6 {
          n324 = xnode ("Register Read")() -> ("Data"=w1125:bool)  [unwired: 1 in, 1 out]
          n325 = local read "LastScan"() -> (w1127:bool)
          n326 = Or(x=w1125, y=w1127) -> (x .or. y?=w1126:bool)
          n327 = case shown="True" w1126 {
            tunnel: w1129 -> [_ w1133]
            tunnel: w1128 -> [_ w1130]
            frame False {
            }
            frame True {
              n328 = while {
                shift-right: [w1137] -> _
                shift-left: w1130 -> [w1142]
                tunnel: fxp<+/-,48,16> 0.0048828125 ("y") -> [w1136]
                stop <- w1138 stop-if-true
                w1135 = fxp<+/-,48,16> 0.0 ("t")
                n329 = xnode "High Throughput Subtract"("x"=w1142, "y"=w1136) -> ("x-y"=w1139:fxp<+/-,48,16>)
                n330 = Less Or Equal To 0?(x=w1139) -> (x <= 0?=w1140:bool)
                n331 = Less Or Equal?(x=w1139, y=w1135) -> (x <= y?=w1141:bool)
                n332 = Select(t=w1135, s=w1140, f=w1139) -> (s? t:f=w1137:fxp<+/-,48,16>)
                n333 = xnode "FPGA I/O Node"("Connector0/AO1"=w1137) -> ()  [unwired: 1 in, 1 out]
                n334 = Compound Arithmetic op=OR(w1140, w1141) -> (w1138:bool)
                n335 = call "Wait14"("Count(uSec)"=u16 100) -> ()  [unwired: 1 out]
              }
              n336 = while {
                shift-right: [w1146] -> _
                shift-left: w1133 -> [w1151]
                tunnel: fxp<+/-,48,16> 0.0048828125 ("y") -> [w1145]
                stop <- w1147 stop-if-true
                w1144 = fxp<+/-,48,16> 0.0 ("t")
                n337 = xnode "High Throughput Subtract"("x"=w1151, "y"=w1145) -> ("x-y"=w1148:fxp<+/-,48,16>)
                n338 = Less Or Equal To 0?(x=w1148) -> (x <= 0?=w1149:bool)
                n339 = Less Or Equal?(x=w1148, y=w1144) -> (x <= y?=w1150:bool)
                n340 = Select(t=w1144, s=w1149, f=w1148) -> (s? t:f=w1146:fxp<+/-,48,16>)
                n341 = xnode "FPGA I/O Node"("Connector0/AO0"=w1146) -> ()  [unwired: 1 in, 1 out]
                n342 = Compound Arithmetic op=OR(w1149, w1150) -> (w1147:bool)
                n343 = call "Wait13"("Count(uSec)"=u16 100) -> ()  [unwired: 1 out]
              }
            }
          }
        }
        frame #7 {
          n344 = call "Wait16"("Count(uSec)"=u8 100) -> ()  [unwired: 1 out]
        }
        frame #8 {
          n345 = local write "ScanFinished?"(TRUE ("ScanFinished?")) -> ()
        }
      }
      n346 = while {
        stop <- w37 stop-if-true
        n347 = xnode ("Register Read")() -> ("Data"=w38:bool)  [unwired: 1 in, 1 out]
        n348 = xnode ("FIFO Method Node")() -> ("Number of Elements to Read"=w36:u32)  [unwired: 1 in, 1 out]
        n349 = local read "ScanFinished?"() -> (w39:bool)
        n350 = call "Wait8"("Count(uSec)"=u8 200 ("Count(mSec)")) -> ()  [unwired: 1 out]
        n351 = Or(x=w39, y=w38) -> (x .or. y?=w37:bool)
        n352 = Greater Than 0?(x=w36) -> (x > 0?=w35:bool)
        n353 = case shown="True" w35 {
          frame False {
          }
          frame True {
            # "push data in swapbuffer from target to host and clear buffer synchronously"
            n354 = flat-sequence {
              frame #0 {
              }
              frame #1 {
                n355 = xnode ("FIFO Method Node")("Timeout"=8192) -> ("Element"=w41:u8)  [unwired: 1 in, 2 out]
                n356 = case shown="0, Default" w41 {
                  frame 0, Default {
                    n357 = flat-sequence {
                      frame #0 {
                        n358 = node-c288(refnum<k21> "8MHz" ("Source Name")) -> (w45:T1)
                        n359 = timed-loop {
                          timing: w45 -> [_]
                          timing-out: [_] -> w44
                          shift-right: [w47] -> _
                          shift-left: _ -> [w54]
                          shift-right: [w54] -> _
                          shift-left: _ -> [w53]
                          shift-right: [w53] -> _
                          shift-left: _ -> [w50]
                          i -> [w46]
                          stop <- w51 stop-if-true
                          n360 = Greater Or Equal?(x=w46, y=16386) -> (x >= y?=w51:bool)
                          n361 = Greater Or Equal?(x=w46, y=3) -> (x >= y?=w49:bool)
                          n362 = case shown="True" w49 {
                            tunnel: w50 -> [_ w55]
                            frame False {
                            }
                            frame True {
                              n363 = xnode ("FIFO Method Node")("Element"=w55, "Timeout"=0) -> ()  [unwired: 1 in, 2 out]
                            }
                          }
                          n364 = xnode ("Memory Method Node")("Address"=w46) -> ("Data"=w47:fxp<+/-,48,16>)  [unwired: 1 in, 1 out]
                        }
                        n365 = node-c288(w44) -> ()
                      }
                      frame #1 {
                        n366 = node-c288() -> (w64:T1)  [unwired: 1 in]
                        n367 = timed-loop {
                          timing: w64 -> [_]
                          timing-out: [_] -> w63
                          i -> [w65]
                          stop <- w66 stop-if-true
                          n368 = xnode ("Memory Method Node")("Address"=w65, "Data"=fxp<+/-,48,16> -100.0) -> ()  [unwired: 1 in, 1 out]
                          n369 = Greater Or Equal?(x=w65, y=16383) -> (x >= y?=w66:bool)
                        }
                        n370 = node-c288(w63) -> ()
                      }
                    }
                  }
                  frame 1 {
                    n371 = flat-sequence {
                      frame #0 {
                        n372 = node-c288(refnum<k21> "8MHz" ("Source Name")) -> (w75:T1)
                        n373 = timed-loop {
                          timing: w75 -> [_]
                          timing-out: [_] -> w74
                          shift-right: [w84] -> _
                          shift-left: _ -> [w83]
                          shift-right: [w83] -> _
                          shift-left: _ -> [w82]
                          shift-right: [w82] -> _
                          shift-left: _ -> [w79]
                          i -> [w78]
                          stop <- w80 stop-if-true
                          n374 = Greater Or Equal?(x=w78, y=3) -> (x >= y?=w77:bool)
                          n375 = Greater Or Equal?(x=w78, y=16386) -> (x >= y?=w80:bool)
                          n376 = case shown="True" w77 {
                            tunnel: w79 -> [_ w85]
                            frame False {
                            }
                            frame True {
                              n377 = xnode ("FIFO Method Node")("Element"=w85, "Timeout"=0) -> ()  [unwired: 1 in, 2 out]
                            }
                          }
                          n378 = xnode ("Memory Method Node")("Address"=w78) -> ("Data"=w84:fxp<+/-,48,16>)  [unwired: 1 in, 1 out]
                        }
                        n379 = node-c288(w74) -> ()
                      }
                      frame #1 {
                        n380 = node-c288() -> (w94:T1)  [unwired: 1 in]
                        n381 = timed-loop {
                          timing: w94 -> [_]
                          timing-out: [_] -> w93
                          i -> [w95]
                          stop <- w97 stop-if-true
                          n382 = xnode ("Memory Method Node")("Address"=w95, "Data"=fxp<+/-,48,16> -100.0) -> ()  [unwired: 1 in, 1 out]
                          n383 = Greater Or Equal?(x=w95, y=16383) -> (x >= y?=w97:bool)
                        }
                        n384 = node-c288(w93) -> ()
                      }
                    }
                  }
                  frame 2 {
                    n385 = flat-sequence {
                      frame #0 {
                        n386 = node-c288(refnum<k21> "8MHz" ("Source Name")) -> (w105:T1)
                        n387 = timed-loop {
                          timing: w105 -> [_]
                          timing-out: [_] -> w104
                          shift-right: [w106] -> _
                          shift-left: _ -> [w114]
                          shift-right: [w114] -> _
                          shift-left: _ -> [w113]
                          shift-right: [w113] -> _
                          shift-left: _ -> [w110]
                          i -> [w107]
                          stop <- w111 stop-if-true
                          n388 = Greater Or Equal?(x=w107, y=3) -> (x >= y?=w109:bool)
                          n389 = Greater Or Equal?(x=w107, y=16386) -> (x >= y?=w111:bool)
                          n390 = case shown="True" w109 {
                            tunnel: w110 -> [_ w115]
                            frame False {
                            }
                            frame True {
                              n391 = xnode ("FIFO Method Node")("Element"=w115, "Timeout"=0) -> ()  [unwired: 1 in, 2 out]
                            }
                          }
                          n392 = xnode ("Memory Method Node")("Address"=w107) -> ("Data"=w106:fxp<+/-,48,16>)  [unwired: 1 in, 1 out]
                        }
                        n393 = node-c288(w104) -> ()
                      }
                      frame #1 {
                        n394 = node-c288() -> (w124:T1)  [unwired: 1 in]
                        n395 = timed-loop {
                          timing: w124 -> [_]
                          timing-out: [_] -> w123
                          i -> [w126]
                          stop <- w127 stop-if-true
                          n396 = xnode ("Memory Method Node")("Address"=w126, "Data"=fxp<+/-,48,16> -100.0) -> ()  [unwired: 1 in, 1 out]
                          n397 = Greater Or Equal?(x=w126, y=16383) -> (x >= y?=w127:bool)
                        }
                        n398 = node-c288(w123) -> ()
                      }
                    }
                  }
                }
              }
              frame #2 {
              }
            }
          }
        }
      }
    }
    frame #4 {
      n399 = local write "TargetDone?"(TRUE ("TargetDone?")) -> ()
    }
  }
